vi "Trajectory_Execution_CREATE_DIFF_POSE_EST.vi"() -> ()   [LabVIEW 2019]
uses:
  <vilib>/Rock Robotics/WPI/ThirdParty/JAS_Junk/TrajLib/Trajectory_Library.lvlib
  <vilib>/Analysis/Matrix/Datatypes/RealMatrix.ctl
  <vilib>/Analysis/Matrix/NI_Matrix.lvlib
panel:
  out "Error":errorcluster
  in  "VisionMeasurementStdDevs":T1=[[0.1], [0.1], [0.01]]
  in  "LocalMeasurementStdDevs":T1=[[0.01], [0.01], [0.001]]
  in  "StateStdDevs":T1=[[0.02], [0.02], [0.01], [0.02], [0.02]]
  # "DIFF DRIVE TRAIN POSE EST CONFIGURATION"
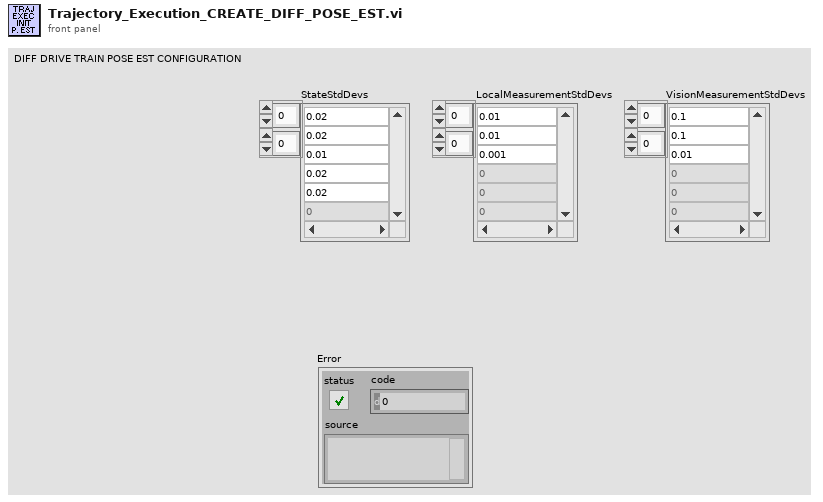
[diagram p1: front panel]
types:
  T1 = typedef "NI_Matrix.lvlib/RealMatrix.ctl" = dbl[][]
  T2 = typedef "Trajectory_Library.lvlib/ROTATION2D.ctl" = cluster{"VALUE":dbl, "COS":dbl, "SIN":dbl}
  T3 = typedef "Trajectory_Library.lvlib/POSE2D.ctl" = cluster{"TRANSLATION":T4, "ROTATION":T2}
  T4 = typedef "Trajectory_Library.lvlib/TRANSLATION2D.ctl" = cluster{"X":dbl, "Y":dbl}
  T5 = typedef "Trajectory_Library.lvlib/DIFF_DRIVE_POSE_EST.ctl" = cluster{"M_VisionContR":T1, "m_nominal_dT":dbl, "m_PrevTime_Sec":dbl, "m_GyroOffset":T2, "m_PrevAngle":T2, "StartLeftEnc_M":dbl, "StartRightEnc_M":dbl, "m_Observer":T6, "Pose_Buffer":T9}
  T6 = typedef "Trajectory_Library.lvlib/UNSCENTED_KALMAN_FILTER.ctl" = cluster{"m_P":T1, "m_xHat":T1, "States":i32, "Outputs":i32, "m_ContR":T1, "m_ContQ":T1, "m_SigmasF":T1, "m_dT_Sec":dbl, "MERWE_SCALED_SIGMA_PTS":T7, "meanFuncX":T8, "meanFuncY":T8, "residualFuncX":T8, "residualFuncY":T8, "addFuncX":T8, "addFuncXExtra":variant, "residualFuncYExtra":variant, "residualFuncXExtra":variant, "MeanFuncYExtra":variant, "MeanFuncXExtra":variant, "Inputs":i32}
  T7 = typedef "Trajectory_Library.lvlib/MERWE_SCALED_SIGMA_PTS.ctl" = cluster{"m_Wm":T1, "States":i32, "Alpha":dbl, "m_Wc":T1, "Kappa":i32}
  T8 = typedef "Trajectory_Library.lvlib/CALLBACK_FUNC_TYPE.ctl" = refnum<vi>
  T9 = typedef "Trajectory_Library.lvlib/TIME_INTERPOLATABLE_POSE2D.ctl" = cluster{"TimeStamps":dbl[], "Pose":T3[], "Min_TimeStamp":dbl, "Max_TimeStamp":dbl, "ItemCount":i32, "MaxBufferTime":dbl}
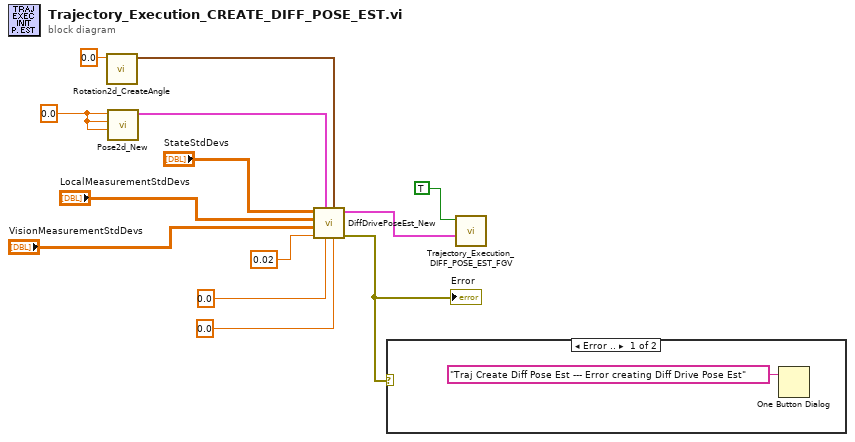
[diagram p0: block diagram]
diagram:
  w2 = 0.0 ("X")
  n1 = call <vilib>:"Rotation2d_CreateAngle.vi"("Angle"=0.0) -> ("ROTATION"=w4:T2)  [unwired: 10 in]
  n2 = call <vilib>:"Pose2d_New.vi"("Heading"=w2, "Y"=w2, "X"=w2) -> ("out POSe"=w3:T3)  [unwired: 8 in]
  n3 = call <vilib>:"DiffDrivePoseEst_New.vi"("RightDistance_M"=0.0, "gyroAngle"=w4, "LeftDistance_M"=0.0, "InitialPose"=w3, "dt_Seconds"=0.02, "VisionMeasurementStdDevs"="VisionMeasurementStdDevs", "LocalMeasurementStdDevs"="LocalMeasurementStdDevs", "StateStdDevs"="StateStdDevs") -> ("Error"=w1:errorcluster, "DiffDrivePoseEstimate"=w6:T5)  [unwired: 2 in]
  "Error" <- w1
  n4 = case shown="Error .." w1 {
    frame Error {
      n5 = One Button Dialog(message="Traj Create Diff Pose Est --- Error creating Diff Drive Pose Est") -> ()  [unwired: 1 in, 1 out]
    }
    frame No Error {
    }
  }
  n6 = call "Trajectory_Execution_DIFF_POSE_EST_FGV.vi"("IN DIFF_DRIVE_POSE_EST"=w6, "WRITE"=TRUE) -> ()  [unwired: 9 in, 1 out]
